vi "ODriveControl.vi"() -> ()   [LabVIEW 2019]
uses:
  <vilib>/Platform/TimedLoop/XDataNode/timing_clust.ctl
  <vilib>/Platform/TimedLoop/XDataNode/nitl_modes.ctl
  <vilib>/Platform/TimedLoop/XDataNode/wakeup.ctl
  8d920558-ab16-4e3c-b164-eadcdcc29f7c.vi
  9b83eaf6-1c06-4c01-825f-3d1d9790e297.vi
  84d8e7d4-34dc-4654-bc51-b5293f88ee83.vi
  <vilib>/Utility/file.llb/Write Delimited Spreadsheet (string).vi
  <vilib>/platform/TimedLoop/XDataNode/XDataNode.xnode
  <vilib>/Platform/TimedLoop/XDataNode/XDNodeRunTimeDep.lvlib
panel:
  in  "?":T1(tab)
  in  "Record":bool
  in  "Initalize":bool
  in  "Enable":bool
  in  "Control Method":enum32{"Velocity", "Torque ", "Position"}(tab)
  in  "Set Motor (Rev/s)":dbl
  in  "Set Torque (NM)":dbl
  in  "Set Position (REV)":dbl
  in  "RPM Limit":dbl
  in  "Current Limit":dbl
  in  "Reboot":bool
  in  "ODrive COM":refnum<visa-resource-name>
  in  "Stop":bool
  in  "?":enum32{"Power Supply"}(tab)
  out "Voltage (V)":dbl
  out "Current (A)":dbl
  out "Power (W)":dbl
  in  "?":enum32{"Motor"}(tab)
  out "RPM":dbl
  out "Position (REV)":dbl
  out "REV/s":dbl
  in  "Motor On/Off":bool
  out "Saving To:":path caption="start path"
  out "Time (s)":dbl
  in  "D Gain":dbl
  in  "I Gain":dbl
  in  "P Gain":dbl
  out "Start Tick":dbl
  out "Write Time":dbl
  out "Motor Spin?":errorcluster
  out "Settings Command":string
  out "ODRIVE Settings":errorcluster
  out "ODRIVE Connect":errorcluster
  out "MotorINT0":errorcluster
  out "Connect?":errorcluster
  out "INTMotor0":string
  out "INTVelMode":string
  in  "Tuner 3":dbl
  in  "Tuner":dbl
  in  "Tuner 4":dbl
  # "ODRIVE Controller"
  # "NEO:\nP: 1.1\nI: 0.08\nD: 0.04"
  # "Instructions for use:\nkfjdklfjsdkj\nfjkdfld;j"
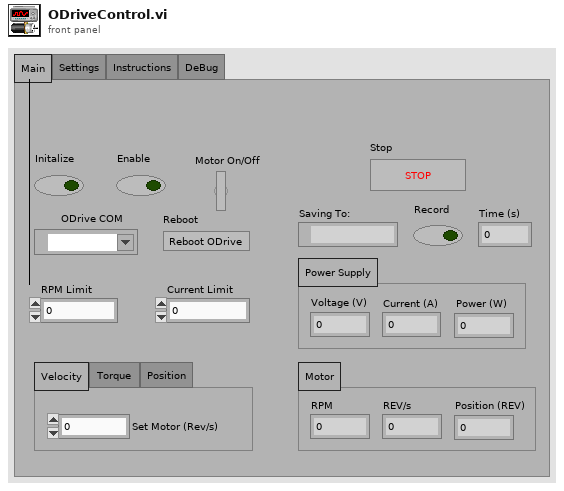
[diagram p1: front panel]
types:
  T1 = enum32{"Main", "Settings", "Instructions", "DeBug"}
  T2 = typedef "XDNodeRunTimeDep.lvlib/timing_clust.ctl" = cluster{"Expected End [f-1]":u64, "Actual End [f-1]":u64, "Finished Late? [f-1]":bool, "Expected End [i-1]":u64, "Actual End [i-1]":u64, "Finished Late? [i-1]":bool, "Expected Start [i]":u64, "Actual Start [i]":u64, "Expected Start [f]":u64, "Actual Start [f]":u64, "Source Name":string, "Structure Name":string, "Period":i64, "Deadline":i64, "Offset":i64, "Start":i64, "Priority":i32, "Timeout":i32, "Mode":T3, "Wakeup Reason":T4, "Error":errorcluster, "Source Type":string, "Secondary Source Type":string, "Global End Time":u64, "Global Start Time":u64, "Frame Duration":u64, "Iteration Duration":u64, "Assigned CPU":i32, "I/O Scan Engine Mode":u32}
  T3 = typedef "XDNodeRunTimeDep.lvlib/nitl_modes.ctl" = enum32{"No Change", "Process missed periods, maintain original phase", "Discard missed periods, maintain original phase", "Process missed periods, ignore original phase", "Discard missed periods, ignore original phase"}
  T4 = typedef "XDNodeRunTimeDep.lvlib/wakeup.ctl" = enum32{"Normal", "Aborted", "Asynchronous wakeup", "Timing source error", "Timed loop error", "Timeout"}
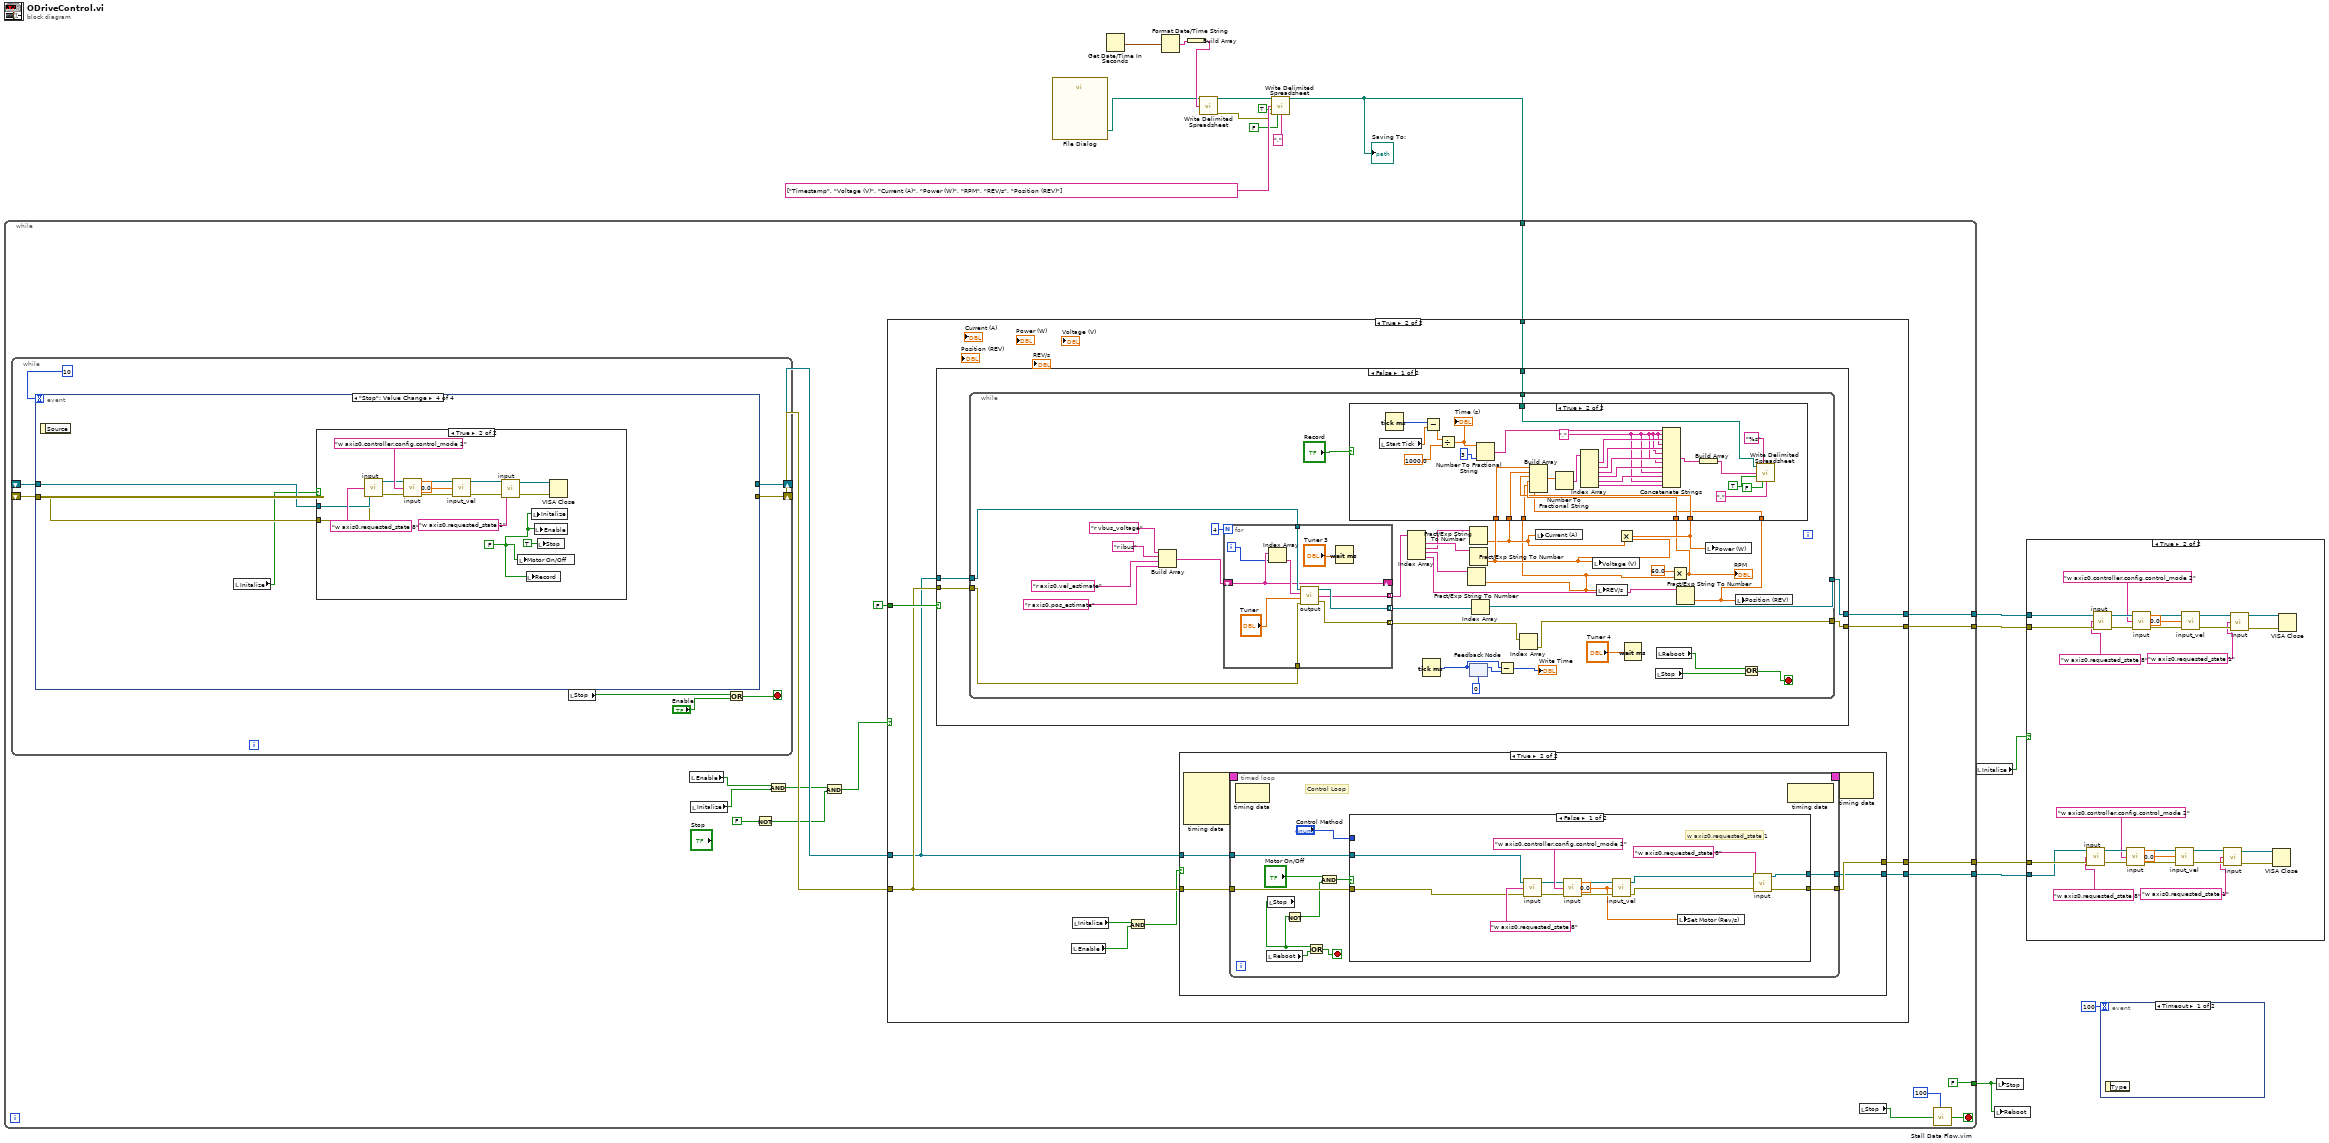
[diagram p0: block diagram]
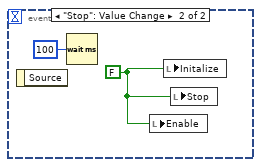
[diagram p2: hidden frame]
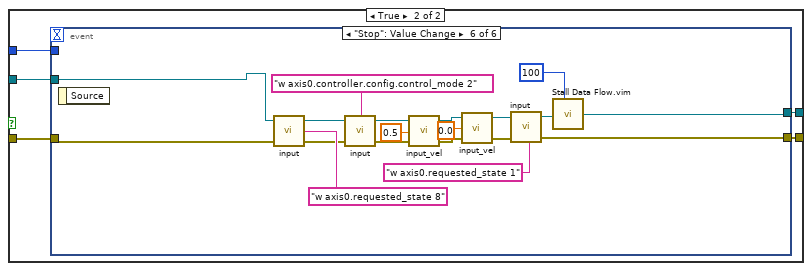
[diagram p6: hidden frame]
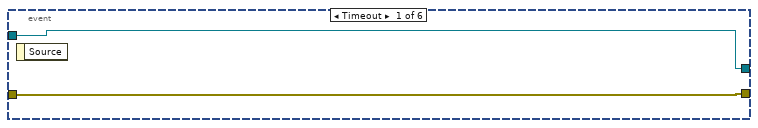
[diagram p7: hidden frame]
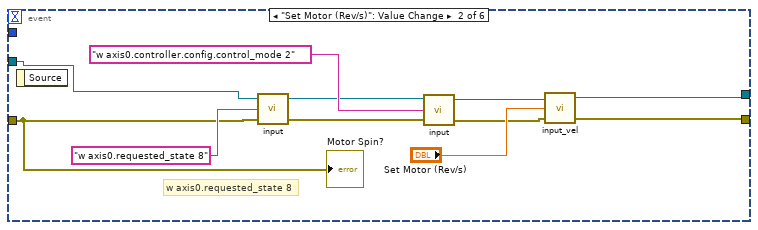
[diagram p8: hidden frame]
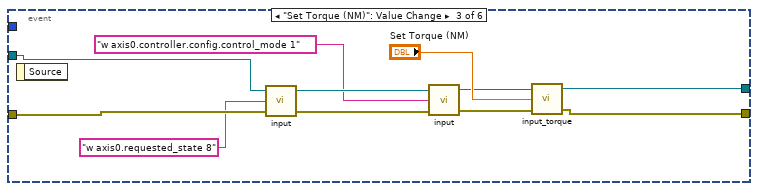
[diagram p9: hidden frame]
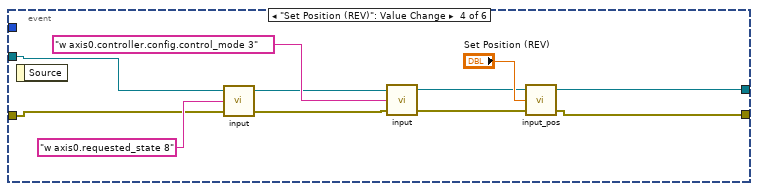
[diagram p10: hidden frame]
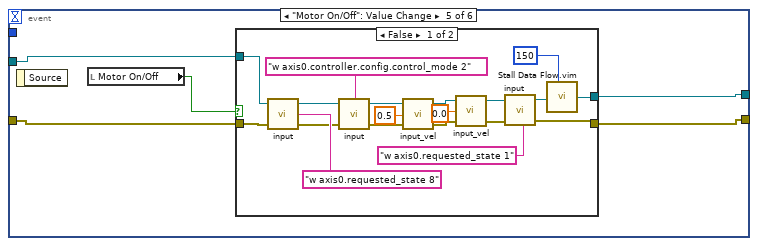
[diagram p11: hidden frame]
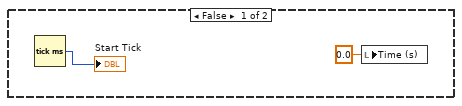
[diagram p13: hidden frame]
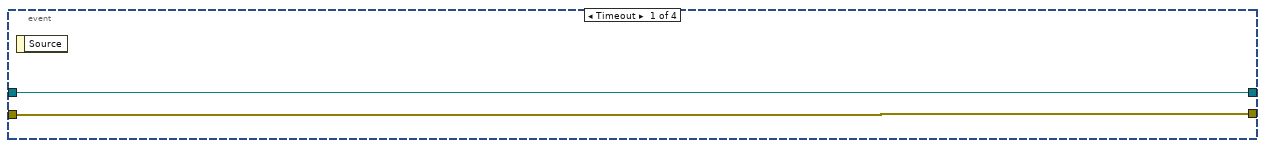
[diagram p15: hidden frame]
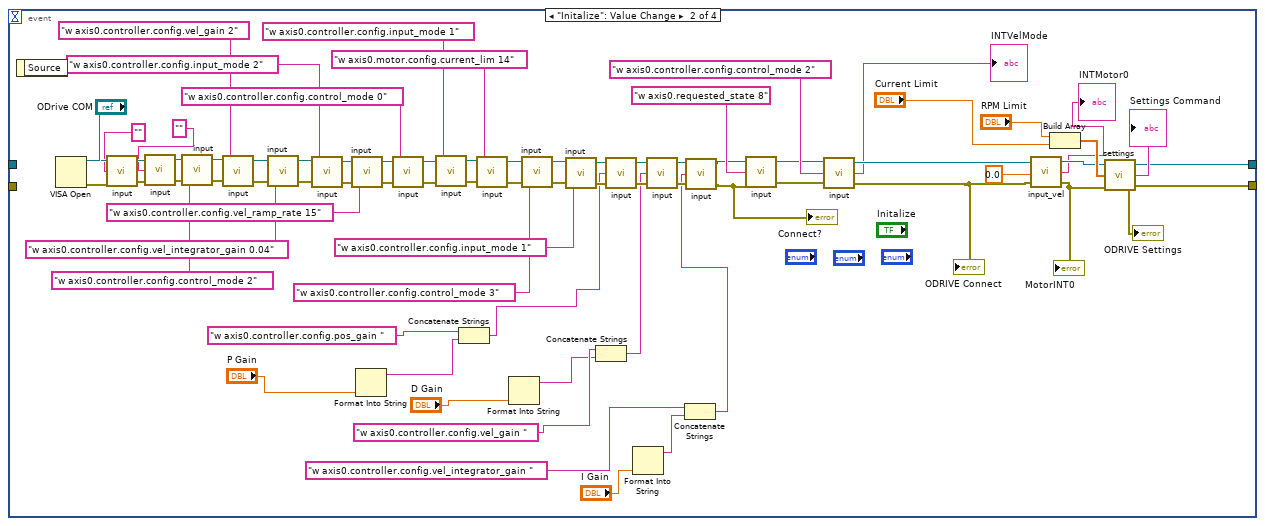
[diagram p16: hidden frame]
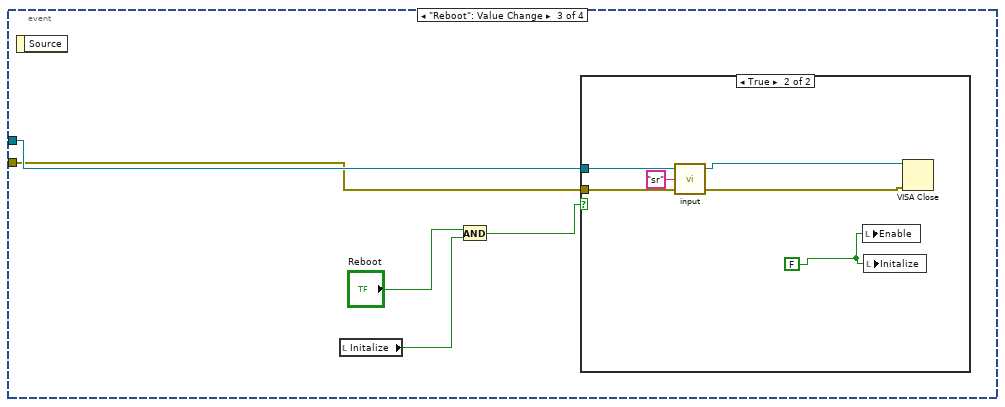
[diagram p17: hidden frame]
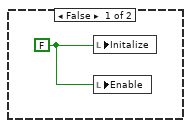
[diagram p19: hidden frame]
diagram:
  n1 = call "File Dialog"() -> ("selected path"=w2:path)  [unwired: 12 in, 3 out]
  n2 = Get Date/Time In Seconds() -> (seconds since 1Jan1904=w6:timestamp)
  n3 = Format Date/Time String(seconds (now)=w6) -> (date/time string=w11:string)  [unwired: 2 in]
  n4 = Build Array(w11) -> (w10:string[])
  n5 = call-poly <vilib>:"Write Delimited Spreadsheet.vi"("file path (dialog if empty)"=w2, "1D data"=w10) -> ("new file path (Not A Path if cancelled)"=w9:path, "error out"=w5:errorcluster)  [unwired: 12 in]
  n6 = call-poly <vilib>:"Write Delimited Spreadsheet.vi"("file path (dialog if empty)"=w9, "1D data"=string[] ["Timestamp", "Voltage (V)", "Current (A)", "Power (W)", "RPM", "REV/s", "Position (REV)"], "append to file? (new file:F)"=TRUE, "error in (no error)"=w5, "transpose? (no:F)"=FALSE, "delimiter (\\t)"="," ("delimiter (\\t)")) -> ("new file path (Not A Path if cancelled)"=w1:path)  [unwired: 8 in, 1 out]
  "Saving To:" <- w1
  n7 = while {
    tunnel: [w32] -> w18
    tunnel: [w31] -> w17
    tunnel: [w30] -> w16
    tunnel: [w29] -> w15
    tunnel: [FALSE] -> w12
    tunnel: w1 -> [w19]
    stop <- w25 stop-if-true
    n8 = while {
      shift-right: [w258] -> w35
      shift-left: _ -> [w260]
      shift-right: [w257] -> w36
      shift-left: _ -> [w259]
      stop <- w256 stop-if-true
      n9 = event shown="[3] \"Stop\": Value Change" {
        selector: _ -> [_ _ _ _]
        dyn-events: _ -> [_ _ _ _]
        timeout: 10 -> [_ _ _ _]
        tunnel: [w262 w321 _ _] -> w257
        tunnel: [w263 w322 _ _] -> w258
        tunnel: w260 -> [w263 _ w342 w351]
        tunnel: w259 -> [w262 _ w341 w350]
        event Timeout {
          n10 = event-data() -> ()  [unwired: 1 in, 1 out]
        }
        event "Initalize": Value Change {
          n11 = event-data() -> ()  [unwired: 1 in, 1 out]
          n12 = VISA Open(VISA resource name="ODrive COM") -> (VISA resource name=w283:refnum<visa-resource-name>, error out=w282:errorcluster)  [unwired: 4 in]
          n13 = call "input.vi"("error in (no error)"=w282, "commando"="", "VISA in"=w283) -> ("error out"=w278:errorcluster, "VISA out"=w280:refnum<visa-resource-name>)  [unwired: 1 out]
          n14 = call "input.vi"("error in (no error)"=w278, "commando"="", "VISA in"=w280) -> ("error out"=w277:errorcluster, "VISA out"=w279:refnum<visa-resource-name>)  [unwired: 1 out]
          n15 = call "input.vi"("error in (no error)"=w277, "commando"="w axis0.controller.config.control_mode 2", "VISA in"=w279) -> ("error out"=w317:errorcluster, "VISA out"=w318:refnum<visa-resource-name>)  [unwired: 1 out]
          n16 = call "input.vi"("error in (no error)"=w317, "commando"="w axis0.controller.config.vel_gain 2", "VISA in"=w318) -> ("error out"=w315:errorcluster, "VISA out"=w316:refnum<visa-resource-name>)  [unwired: 1 out]
          n17 = call "input.vi"("error in (no error)"=w315, "commando"="w axis0.controller.config.vel_integrator_gain 0.04", "VISA in"=w316) -> ("error out"=w313:errorcluster, "VISA out"=w314:refnum<visa-resource-name>)  [unwired: 1 out]
          n18 = call "input.vi"("error in (no error)"=w313, "commando"="w axis0.controller.config.input_mode 2", "VISA in"=w314) -> ("error out"=w311:errorcluster, "VISA out"=w312:refnum<visa-resource-name>)  [unwired: 1 out]
          n19 = call "input.vi"("error in (no error)"=w311, "commando"="w axis0.controller.config.vel_ramp_rate 15", "VISA in"=w312) -> ("error out"=w309:errorcluster, "VISA out"=w310:refnum<visa-resource-name>)  [unwired: 1 out]
          n20 = Format Into String("P Gain") -> (resulting string=w273:string)  [unwired: 3 in, 1 out]
          n21 = call "input.vi"("error in (no error)"=w309, "commando"="w axis0.controller.config.control_mode 0", "VISA in"=w310) -> ("error out"=w293:errorcluster, "VISA out"=w294:refnum<visa-resource-name>)  [unwired: 1 out]
          n22 = call "input.vi"("error in (no error)"=w293, "commando"="w axis0.controller.config.input_mode 1", "VISA in"=w294) -> ("error out"=w303:errorcluster, "VISA out"=w304:refnum<visa-resource-name>)  [unwired: 1 out]
          n23 = Concatenate Strings("w axis0.controller.config.pos_gain " ("commando"), w273) -> (w272:string)
          n24 = call "input.vi"("error in (no error)"=w303, "commando"="w axis0.motor.config.current_lim 14", "VISA in"=w304) -> ("error out"=w301:errorcluster, "VISA out"=w302:refnum<visa-resource-name>)  [unwired: 1 out]
          n25 = Format Into String("D Gain") -> (resulting string=w269:string)  [unwired: 3 in, 1 out]
          n26 = call "input.vi"("error in (no error)"=w301, "commando"="w axis0.controller.config.control_mode 3", "VISA in"=w302) -> ("error out"=w299:errorcluster, "VISA out"=w300:refnum<visa-resource-name>)  [unwired: 1 out]
          n27 = call "input.vi"("error in (no error)"=w299, "commando"="w axis0.controller.config.input_mode 1", "VISA in"=w300) -> ("error out"=w297:errorcluster, "VISA out"=w298:refnum<visa-resource-name>)  [unwired: 1 out]
          n28 = Concatenate Strings("w axis0.controller.config.vel_gain " ("commando"), w269) -> (w268:string)
          n29 = call "input.vi"("error in (no error)"=w297, "commando"=w272, "VISA in"=w298) -> ("error out"=w295:errorcluster, "VISA out"=w296:refnum<visa-resource-name>)  [unwired: 1 out]
          n30 = Format Into String("I Gain") -> (resulting string=w266:string)  [unwired: 3 in, 1 out]
          n31 = call "input.vi"("error in (no error)"=w295, "commando"=w268, "VISA in"=w296) -> ("error out"=w291:errorcluster, "VISA out"=w292:refnum<visa-resource-name>)  [unwired: 1 out]
          n32 = Concatenate Strings("w axis0.controller.config.vel_integrator_gain " ("commando"), w266) -> (w264:string)
          n33 = call "input.vi"("error in (no error)"=w291, "commando"=w264, "VISA in"=w292) -> ("error out"=w284:errorcluster, "VISA out"=w285:refnum<visa-resource-name>)  [unwired: 1 out]
          "Connect?" <- w284
          n34 = call "input.vi"("error in (no error)"=w284, "commando"="w axis0.requested_state 8", "VISA in"=w285) -> ("error out"=w324:errorcluster, "VISA out"=w325:refnum<visa-resource-name>)  [unwired: 1 out]
          n35 = call "input.vi"("error in (no error)"=w324, "commando"="w axis0.controller.config.control_mode 2", "VISA in"=w325) -> ("error out"=w328:errorcluster, "DEBUG"=→"INTVelMode":string, "VISA out"=w327:refnum<visa-resource-name>)
          "ODRIVE Connect" <- w328
          n36 = call "input_vel.vi"("error in (no error)"=w328, "input"=0.0, "odrive"=w327) -> ("error out"=w331:errorcluster, "String"=→"INTMotor0":string, "VISA resource name out"=w333:refnum<visa-resource-name>)
          "MotorINT0" <- w331
          n37 = Build Array("RPM Limit", "Current Limit") -> (w337:dbl[])
          n38 = call "settings.vi"("error in (no error)"=w331, "values"=w337, "sturing in"=w333) -> ("error out"=w321:errorcluster, "String"=→"Settings Command":string, "sturing out"=w322:refnum<visa-resource-name>)
          "ODRIVE Settings" <- w321
        }
        event "Reboot": Value Change {
          n39 = event-data() -> ()  [unwired: 1 in, 1 out]
          n40 = local read "Initalize"() -> (w340:bool)
          n41 = And(x="Reboot", y=w340) -> (x .and. y?=w338:bool)
          n42 = case shown="True" w338 {
            tunnel: w342 -> [_ w348]
            tunnel: w341 -> [_ w347]
            frame False {
            }
            frame True {
              w343 = FALSE
              n43 = call "input.vi"("error in (no error)"=w347, "commando"="sr", "VISA in"=w348) -> ("error out"=w345:errorcluster, "VISA out"=w344:refnum<visa-resource-name>)  [unwired: 1 out]
              n44 = local write "Enable"(w343) -> ()
              n45 = local write "Initalize"(w343) -> ()
              n46 = VISA Close(VISA resource name=w344, error in (no error)=w345) -> ()  [unwired: 1 out]
            }
          }
        }
        event "Stop": Value Change {
          n47 = event-data() -> ()  [unwired: 1 in, 1 out]
          n48 = local read "Initalize"() -> (w349:bool)
          n49 = case shown="True" w349 {
            tunnel: w351 -> [_ w356]
            tunnel: w350 -> [_ w355]
            frame False {
              w352 = FALSE
              n50 = local write "Initalize"(w352) -> ()
              n51 = local write "Enable"(w352) -> ()
            }
            frame True {
              w353 = FALSE
              n52 = call "input.vi"("error in (no error)"=w355, "commando"="w axis0.requested_state 8", "VISA in"=w356) -> ("error out"=w366:errorcluster, "VISA out"=w363:refnum<visa-resource-name>)  [unwired: 1 out]
              n53 = call "input.vi"("error in (no error)"=w366, "commando"="w axis0.controller.config.control_mode 2", "VISA in"=w363) -> ("error out"=w365:errorcluster, "VISA out"=w364:refnum<visa-resource-name>)  [unwired: 1 out]
              n54 = call "input_vel.vi"("error in (no error)"=w365, "input"=0.0, "odrive"=w364) -> ("error out"=w360:errorcluster, "VISA resource name out"=w361:refnum<visa-resource-name>)  [unwired: 1 out]
              n55 = call "input.vi"("error in (no error)"=w360, "commando"="w axis0.requested_state 1", "VISA in"=w361) -> ("error out"=w357:errorcluster, "VISA out"=w358:refnum<visa-resource-name>)  [unwired: 1 out]
              n56 = local write "Motor On/Off"(w353) -> ()
              n57 = local write "Record"(w353) -> ()
              n58 = local write "Initalize"(w353) -> ()
              n59 = local write "Enable"(w353) -> ()
              n60 = local write "Stop"(TRUE ("Stop")) -> ()
              n61 = VISA Close(VISA resource name=w358, error in (no error)=w357) -> ()  [unwired: 1 out]
            }
          }
        }
      }
      n62 = local read "Stop"() -> (w254:bool)
      n63 = Or(x=w254, y="Enable") -> (x .or. y?=w256:bool)
    }
    n64 = local read "Enable"() -> (w34:bool)
    n65 = local read "Initalize"() -> (w33:bool)
    n66 = Not(x=FALSE) -> (.not. x?=w27:bool)
    n67 = And(x=w34, y=w33) -> (x .and. y?=w28:bool)
    n68 = And(x=w28, y=w27) -> (x .and. y?=w26:bool)
    n69 = case shown="True" w26 {
      tunnel: FALSE ("Reboot") -> [_ w49]
      tunnel: w36 -> [w38 w48]
      tunnel: w35 -> [w37 w47]
      tunnel: [w38 w46] -> w32
      tunnel: [w37 w45] -> w31
      tunnel: [w38 w44] -> w30
      tunnel: [w37 w43] -> w29
      tunnel: w19 -> [_ w39]
      frame False {
      }
      frame True {
        n70 = case shown="False" w49 {
          tunnel: w47 -> [w176 w253]
          tunnel: w48 -> [w175 w252]
          tunnel: [w174 w252] -> w46
          tunnel: [w173 w253] -> w45
          tunnel: w39 -> [w172 _]
          frame False {
            n71 = while {
              tunnel: w176 -> [w206]
              tunnel: w175 -> [w205]
              tunnel: [w202] -> w173
              tunnel: [w201] -> w174
              tunnel: w172 -> [w187]
              stop <- w192 stop-if-true
              n72 = Build Array("r vbus_voltage" ("commando"), "r ibus" ("commando"), "r axis0.vel_estimate" ("commando"), "r axis0.pos_estimate" ("commando")) -> (w197:string[])
              n73 = for {
                N: 4 -> [_]
                tunnel: w206 -> [w248]
                tunnel: w205 -> [w249]
                tunnel: [w251] -> w204 mode=indexing
                tunnel: [w250] -> w203 mode=indexing
                shift-right: [w244] -> _
                shift-left: w197 -> [w244]
                tunnel: [w243] -> w188 mode=indexing
                i -> [w242]
                n74 = Index Array(array=w244, index=w242) -> (element=w245:string)
                n75 = call "output.vi"("error in (no error)"=w249, "Tuner"="Tuner", "commando"=w245, "VISA in"=w248) -> ("error out"=w250:errorcluster, "Output"=w243:string, "VISA out"=w251:refnum<visa-resource-name>)
                n76 = Wait (ms)(milliseconds to wait="Tuner 3") -> ()  [unwired: 1 out]
              }
              n77 = Index Array(array=w188) -> (element #1=w186:string, element #2=w185:string, element #3=w182:string, element #4=w181:string)  [unwired: 4 in]
              n78 = Tick Count (ms)() -> (millisecond timer value=w194:u32)
              n79 = Fract/Exp String To Number(string=w182) -> (number=w178:dbl)  [unwired: 3 in, 1 out]
              n80 = Fract/Exp String To Number(string=w185) -> (number=w179:dbl)  [unwired: 3 in, 1 out]
              n81 = Fract/Exp String To Number(string=w186) -> (number=w180:dbl)  [unwired: 3 in, 1 out]
              n82 = feedback-in #1(w194) -> ()
              n83 = feedback #1(u32 0 ("millisecond timer value")) -> (w195:u32)
              n84 = Index Array(array=w204) -> (element=w202:refnum<visa-resource-name>)  [unwired: 1 in]
              n85 = Subtract(x=w194, y=w195) -> (x-y=→"Write Time":u32)
              n86 = Index Array(array=w203) -> (element=w201:errorcluster)  [unwired: 1 in]
              n87 = local write "Current (A)"(w179) -> ()
              n88 = local write "Voltage (V)"(w180) -> ()
              n89 = local write "REV/s"(w178) -> ()
              n90 = Multiply(x=w179, y=w180) -> (x*y=w184:dbl)
              n91 = Wait (ms)(milliseconds to wait="Tuner 4") -> ()  [unwired: 1 out]
              n92 = local read "Stop"() -> (w191:bool)
              n93 = local read "Reboot"() -> (w190:bool)
              n94 = Multiply(x=60.0, y=w178) -> (x*y=w183:dbl)
              "RPM" <- w183
              n95 = Fract/Exp String To Number(string=w181) -> (number=w177:dbl)  [unwired: 3 in, 1 out]
              n96 = case shown="True" "Record" {
                tunnel: w187 -> [_ w227]
                tunnel: w184 -> [_ w240]
                tunnel: w183 -> [_ w241]
                tunnel: w180 -> [_ w238]
                tunnel: w179 -> [_ w239]
                tunnel: w178 -> [_ w237]
                tunnel: w177 -> [_ w236]
                frame False {
                  n97 = Tick Count (ms)() -> (millisecond timer value=→"Start Tick":u32)
                  n98 = local write "Time (s)"(0.0 ("Time (s)")) -> ()
                }
                frame True {
                  w215 = "," ("string")
                  n99 = local read "Start Tick"() -> (w233:dbl)
                  n100 = Tick Count (ms)() -> (millisecond timer value=w234:u32)
                  n101 = Subtract(x=w234, y=w233) -> (x-y=w235:dbl)
                  n102 = Divide(x=w235, y=1000.0) -> (x/y=w231:dbl)
                  "Time (s)" <- w231
                  n103 = Number To Fractional String(number=w231, precision (6)=i16 3 ("width (-)")) -> (F-format string=w222:string)  [unwired: 2 in]
                  n104 = Build Array(w238, w239, w240, w241, w237, w236) -> (w224:dbl[])
                  n105 = Number To Fractional String(number=w224) -> (F-format string=w223:string[])  [unwired: 3 in]
                  n106 = Index Array(array=w223) -> (element #1=w221:string, element #2=w220:string, element #3=w219:string, element #4=w217:string, element #5=w216:string, element #6=w218:string)  [unwired: 6 in]
                  n107 = Concatenate Strings(w222, w215, w221, w215, w220, w215, w219, w215, w217, w215, w216, w215, w218) -> (w214:string)
                  n108 = Build Array(w214) -> (w213:string[])
                  n109 = call-poly <vilib>:"Write Delimited Spreadsheet.vi"("file path (dialog if empty)"=w227, "format (%s)"="%s", "1D data"=w213, "append to file? (new file:F)"=TRUE, "transpose? (no:F)"=FALSE, "delimiter (\\t)"="," ("delimiter (\\t)")) -> ()  [unwired: 8 in, 2 out]
                }
              }
              n110 = local write "Power (W)"(w184) -> ()
              n111 = local write "Position (REV)"(w177) -> ()
              n112 = Or(x=w190, y=w191) -> (x .or. y?=w192:bool)
            }
          }
          frame True {
          }
        }
        n113 = local read "Enable"() -> (w41:bool)
        n114 = local read "Initalize"() -> (w42:bool)
        n115 = And(x=w42, y=w41) -> (x .and. y?=w40:bool)
        n116 = case shown="True" w40 {
          tunnel: w48 -> [w50 w55]
          tunnel: w47 -> [w51 w54]
          tunnel: [w50 w53] -> w44
          tunnel: [w51 w52] -> w43
          frame False {
          }
          frame True {
            n117 = node-c288() -> (w57:T2)  [unwired: 4 in]
            n118 = timed-loop {
              timing: w57 -> [_]
              timing-out: [_] -> w56
              tunnel: w54 -> [w67]
              tunnel: [w66] -> w52
              tunnel: [w65] -> w53
              tunnel: w55 -> [w64]
              stop <- w60 stop-if-true
              # "Control Loop"
              n119 = node-c288() -> ()  [unwired: 1 in, 1 out]
              n120 = local read "Reboot"() -> (w59:bool)
              n121 = local read "Stop"() -> (w58:bool)
              n122 = Not(x=w58) -> (.not. x?=w63:bool)
              n123 = Or(x=w58, y=w59) -> (x .or. y?=w60:bool)
              n124 = And(x="Motor On/Off", y=w63) -> (x .and. y?=w62:bool)
              n125 = case shown="False" w62 {
                tunnel: "Control Method" -> [_ w87]
                tunnel: w67 -> [w75 w86]
                tunnel: [w70 w85] -> w66
                tunnel: [w69 w84] -> w65
                tunnel: w64 -> [w76 w83]
                frame False {
                  w74 = 0.0 ("input")
                  # "w axis0.requested_state 1"
                  n126 = call "input.vi"("error in (no error)"=w76, "commando"="w axis0.requested_state 8", "VISA in"=w75) -> ("error out"=w80:errorcluster, "VISA out"=w77:refnum<visa-resource-name>)  [unwired: 1 out]
                  n127 = call "input.vi"("error in (no error)"=w80, "commando"="w axis0.controller.config.control_mode 2", "VISA in"=w77) -> ("error out"=w79:errorcluster, "VISA out"=w78:refnum<visa-resource-name>)  [unwired: 1 out]
                  n128 = call "input_vel.vi"("error in (no error)"=w79, "input"=w74, "odrive"=w78) -> ("error out"=w71:errorcluster, "VISA resource name out"=w72:refnum<visa-resource-name>)  [unwired: 1 out]
                  n129 = local write "Set Motor (Rev/s)"(w74) -> ()
                  n130 = call "input.vi"("error in (no error)"=w71, "commando"="w axis0.requested_state 8", "VISA in"=w72) -> ("error out"=w69:errorcluster, "VISA out"=w70:refnum<visa-resource-name>)  [unwired: 1 out]
                }
                frame True {
                  n131 = event shown="[5] \"Stop\": Value Change" {
                    selector: _ -> [_ _ _ _ _ _]
                    dyn-events: _ -> [_ _ _ _ _ _]
                    timeout: _ -> [_ _ _ _ _ _]
                    tunnel: w87 -> [_ _ _ _ _ _]
                    tunnel: w86 -> [w89 w92 w103 w113 w127 w152]
                    tunnel: [w89 w98 w109 w121 w125 w150] -> w85
                    tunnel: [w88 w99 w110 w120 w124 w149] -> w84
                    tunnel: w83 -> [w88 w93 w102 w112 w126 w151]
                    event Timeout {
                      n132 = event-data() -> ()  [unwired: 1 in, 1 out]
                    }
                    event "Set Motor (Rev/s)": Value Change {
                      # "w axis0.requested_state 8"
                      n133 = event-data() -> ()  [unwired: 1 in, 1 out]
                      n134 = call "input.vi"("error in (no error)"=w93, "commando"="w axis0.requested_state 8", "VISA in"=w92) -> ("error out"=w90:errorcluster, "VISA out"=w91:refnum<visa-resource-name>)  [unwired: 1 out]
                      n135 = call "input.vi"("error in (no error)"=w90, "commando"="w axis0.controller.config.control_mode 2", "VISA in"=w91) -> ("error out"=w95:errorcluster, "VISA out"=w96:refnum<visa-resource-name>)  [unwired: 1 out]
                      n136 = call "input_vel.vi"("error in (no error)"=w95, "input"="Set Motor (Rev/s)", "odrive"=w96) -> ("error out"=w99:errorcluster, "VISA resource name out"=w98:refnum<visa-resource-name>)  [unwired: 1 out]
                      "Motor Spin?" <- w93
                    }
                    event "Set Torque (NM)": Value Change {
                      n137 = event-data() -> ()  [unwired: 1 in, 1 out]
                      n138 = call "input.vi"("error in (no error)"=w102, "commando"="w axis0.requested_state 8", "VISA in"=w103) -> ("error out"=w107:errorcluster, "VISA out"=w108:refnum<visa-resource-name>)  [unwired: 1 out]
                      n139 = call "input.vi"("error in (no error)"=w107, "commando"="w axis0.controller.config.control_mode 1", "VISA in"=w108) -> ("error out"=w104:errorcluster, "VISA out"=w105:refnum<visa-resource-name>)  [unwired: 1 out]
                      n140 = call "input_torque.vi"("error in (no error)"=w104, "input"="Set Torque (NM)", "odrive"=w105) -> ("error out"=w110:errorcluster, "VISA resource name out"=w109:refnum<visa-resource-name>)  [unwired: 1 in]
                    }
                    event "Set Position (REV)": Value Change {
                      n141 = event-data() -> ()  [unwired: 1 in, 1 out]
                      n142 = call "input.vi"("error in (no error)"=w112, "commando"="w axis0.requested_state 8", "VISA in"=w113) -> ("error out"=w114:errorcluster, "VISA out"=w115:refnum<visa-resource-name>)  [unwired: 1 out]
                      n143 = call "input.vi"("error in (no error)"=w114, "commando"="w axis0.controller.config.control_mode 3", "VISA in"=w115) -> ("error out"=w116:errorcluster, "VISA out"=w117:refnum<visa-resource-name>)  [unwired: 1 out]
                      n144 = call "input_pos.vi"("error in (no error)"=w116, "positie"="Set Position (REV)", "VISA in"=w117) -> ("error out"=w120:errorcluster, "VISA out"=w121:refnum<visa-resource-name>)  [unwired: 1 in]
                    }
                    event "Motor On/Off": Value Change {
                      n145 = event-data() -> ()  [unwired: 1 in, 1 out]
                      n146 = local read "Motor On/Off"() -> (w123:bool)
                      n147 = case shown="False" w123 {
                        tunnel: w127 -> [w141 w147]
                        tunnel: w126 -> [w140 w148]
                        tunnel: [w129 w147] -> w125
                        tunnel: [w137 w148] -> w124
                        frame False {
                          n148 = call "input.vi"("error in (no error)"=w140, "commando"="w axis0.requested_state 8", "VISA in"=w141) -> ("error out"=w144:errorcluster, "VISA out"=w143:refnum<visa-resource-name>)  [unwired: 1 out]
                          n149 = call "input.vi"("error in (no error)"=w144, "commando"="w axis0.controller.config.control_mode 2", "VISA in"=w143) -> ("error out"=w133:errorcluster, "VISA out"=w134:refnum<visa-resource-name>)  [unwired: 1 out]
                          n150 = call "input_vel.vi"("error in (no error)"=w133, "input"=0.5, "odrive"=w134) -> ("error out"=w132:errorcluster, "VISA resource name out"=w131:refnum<visa-resource-name>)  [unwired: 1 out]
                          n151 = call "input_vel.vi"("error in (no error)"=w132, "input"=0.0, "odrive"=w131) -> ("error out"=w138:errorcluster, "VISA resource name out"=w139:refnum<visa-resource-name>)  [unwired: 1 out]
                          n152 = call "input.vi"("error in (no error)"=w138, "commando"="w axis0.requested_state 1", "VISA in"=w139) -> ("error out"=w137:errorcluster, "VISA out"=w130:refnum<visa-resource-name>)  [unwired: 1 out]
                          n153 = call "Stall Data Flow.vim"("value in"=w130, "milliseconds to wait"=u32 150) -> ("value out"=w129:refnum<visa-resource-name>)  [unwired: 1 out]
                        }
                        frame True {
                        }
                      }
                    }
                    event "Stop": Value Change {
                      n154 = event-data() -> ()  [unwired: 1 in, 1 out]
                      n155 = call "input.vi"("error in (no error)"=w151, "commando"="w axis0.requested_state 8", "VISA in"=w152) -> ("error out"=w165:errorcluster, "VISA out"=w164:refnum<visa-resource-name>)  [unwired: 1 out]
                      n156 = call "input.vi"("error in (no error)"=w165, "commando"="w axis0.controller.config.control_mode 2", "VISA in"=w164) -> ("error out"=w157:errorcluster, "VISA out"=w158:refnum<visa-resource-name>)  [unwired: 1 out]
                      n157 = call "input_vel.vi"("error in (no error)"=w157, "input"=0.5, "odrive"=w158) -> ("error out"=w156:errorcluster, "VISA resource name out"=w155:refnum<visa-resource-name>)  [unwired: 1 out]
                      n158 = call "input_vel.vi"("error in (no error)"=w156, "input"=0.0, "odrive"=w155) -> ("error out"=w161:errorcluster, "VISA resource name out"=w162:refnum<visa-resource-name>)  [unwired: 1 out]
                      n159 = call "input.vi"("error in (no error)"=w161, "commando"="w axis0.requested_state 1", "VISA in"=w162) -> ("error out"=w149:errorcluster, "VISA out"=w154:refnum<visa-resource-name>)  [unwired: 1 out]
                      n160 = call "Stall Data Flow.vim"("value in"=w154, "milliseconds to wait"=u32 100) -> ("value out"=w150:refnum<visa-resource-name>)  [unwired: 1 out]
                    }
                  }
                }
              }
              n161 = node-c288() -> ()  [unwired: 1 in, 1 out]
            }
            n162 = node-c288(w56) -> ()  [unwired: 1 out]
          }
        }
      }
    }
    n163 = local read "Stop"() -> (w24:bool)
    n164 = call "Stall Data Flow.vim"("value in"=w24, "milliseconds to wait"=u32 100) -> ("value out"=w25:bool)  [unwired: 1 out]
  }
  n165 = local read "Initalize"() -> (w14:bool)
  n166 = local write "Reboot"(w12) -> ()
  n167 = local write "Stop"(w12) -> ()
  n168 = case shown="True" w14 {
    tunnel: w18 -> [_ w387]
    tunnel: w17 -> [_ w385]
    tunnel: w16 -> [_ w373]
    tunnel: w15 -> [_ w371]
    frame False {
    }
    frame True {
      n169 = call "input.vi"("error in (no error)"=w373, "commando"="w axis0.requested_state 8", "VISA in"=w371) -> ("error out"=w375:errorcluster, "VISA out"=w378:refnum<visa-resource-name>)  [unwired: 1 out]
      n170 = call "input.vi"("error in (no error)"=w387, "commando"="w axis0.requested_state 8", "VISA in"=w385) -> ("error out"=w389:errorcluster, "VISA out"=w392:refnum<visa-resource-name>)  [unwired: 1 out]
      n171 = call "input.vi"("error in (no error)"=w375, "commando"="w axis0.controller.config.control_mode 2", "VISA in"=w378) -> ("error out"=w376:errorcluster, "VISA out"=w377:refnum<visa-resource-name>)  [unwired: 1 out]
      n172 = call "input.vi"("error in (no error)"=w389, "commando"="w axis0.controller.config.control_mode 2", "VISA in"=w392) -> ("error out"=w390:errorcluster, "VISA out"=w391:refnum<visa-resource-name>)  [unwired: 1 out]
      n173 = call "input_vel.vi"("error in (no error)"=w376, "input"=0.0, "odrive"=w377) -> ("error out"=w380:errorcluster, "VISA resource name out"=w379:refnum<visa-resource-name>)  [unwired: 1 out]
      n174 = call "input_vel.vi"("error in (no error)"=w390, "input"=0.0, "odrive"=w391) -> ("error out"=w394:errorcluster, "VISA resource name out"=w393:refnum<visa-resource-name>)  [unwired: 1 out]
      n175 = call "input.vi"("error in (no error)"=w380, "commando"="w axis0.requested_state 1", "VISA in"=w379) -> ("error out"=w382:errorcluster, "VISA out"=w381:refnum<visa-resource-name>)  [unwired: 1 out]
      n176 = call "input.vi"("error in (no error)"=w394, "commando"="w axis0.requested_state 1", "VISA in"=w393) -> ("error out"=w396:errorcluster, "VISA out"=w395:refnum<visa-resource-name>)  [unwired: 1 out]
      n177 = VISA Close(VISA resource name=w381, error in (no error)=w382) -> ()  [unwired: 1 out]
      n178 = VISA Close(VISA resource name=w395, error in (no error)=w396) -> ()  [unwired: 1 out]
    }
  }
  n179 = event shown="[0] Timeout" {
    selector: _ -> [_ _]
    dyn-events: _ -> [_ _]
    timeout: 100 -> [_ _]
    event Timeout {
      n180 = event-data() -> ()  [unwired: 1 in, 1 out]
    }
    event "Stop": Value Change {
      w397 = FALSE
      n181 = event-data() -> ()  [unwired: 1 in, 1 out]
      n182 = Wait (ms)(milliseconds to wait=u32 100) -> ()  [unwired: 1 out]
      n183 = local write "Enable"(w397) -> ()
      n184 = local write "Initalize"(w397) -> ()
      n185 = local write "Stop"(w397) -> ()
    }
  }
